vi "NGTS_DAQmx Analog Channel Scale Calibration.vi"(0 "Scale Identifier":string="Test Cal", 1 "scaled min":dbl=5.0, 2 "scaled max":dbl=1.0, 3 "scaled units":string="psi", 4 "prescaled units":string="Amps", 5 "error in":errorcluster, 6 "prescaled min":dbl=5.0, 7 "Save As Global Channel":bool, 8 "prescaled max":dbl=1.0, 9 "Author":string="Mike Ashe") -> (14 "Custom Scale Out":tag, 19 "error out":errorcluster)   [LabVIEW 2018]
doc: "Creates a new custom scale using the \"Map Ranges\" version of the \"DAQmx Create Scale (Version).vi\". It first deletes any saved scale of the same name. The Mapped Range is from Prescaled Min & Max to Scaled Min & Max. When using this method, values outside the scaled range are clipped on reads and generate an error on writes. It optionally saves the new scale to MAX.\n\nCurrently only Volts and Amps are used as Prescaled Units. \n\n2007-11 Mike Ashe\nmichael.ashe@imaginatics.net\nCell: 860-961-0876"
uses:
  <vilib>/DAQmx/create/scale.llb/DAQmx Create Scale (Linear).vi
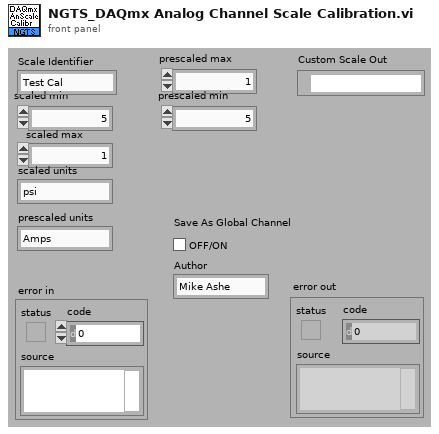
[diagram p1: front panel]
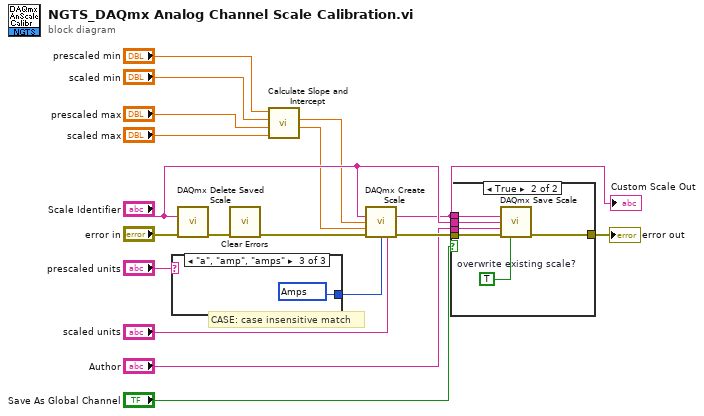
[diagram p0: block diagram]
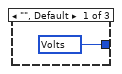
[diagram p2: hidden frame]
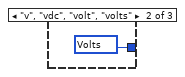
[diagram p3: hidden frame]
diagram:
  # "CASE: case insensitive match"
  n1 = case shown="\"a\", \"amp\", \"amps\"" "prescaled units" {
    tunnel: [w19 w20 w21] -> w10
    frame "", Default {
      w19 = 10348 items=["Volts"=10348, "Amps"=10342, "Deg F"=10144, "Deg C"=10143, "Deg R"=10145, "Kelvins"=10325, "Strain"=10299, "Ohms"=10384, "Hz"=10373, "Seconds"=10364, "Meters"=10219, "Inches"=10379, "Degrees"=10146, "Radians"=10273, "g"=10186, "m/s^2"=12470, "Pascals"=10081, "From TEDS"=12516] ("pre-scaled units")
    }
    frame "v", "vdc", "volt", "volts" {
      w20 = 10348 items=["Volts"=10348, "Amps"=10342, "Deg F"=10144, "Deg C"=10143, "Deg R"=10145, "Kelvins"=10325, "Strain"=10299, "Ohms"=10384, "Hz"=10373, "Seconds"=10364, "Meters"=10219, "Inches"=10379, "Degrees"=10146, "Radians"=10273, "g"=10186, "m/s^2"=12470, "Pascals"=10081, "From TEDS"=12516] ("pre-scaled units")
    }
    frame "a", "amp", "amps" {
      w21 = 10342 items=["Volts"=10348, "Amps"=10342, "Deg F"=10144, "Deg C"=10143, "Deg R"=10145, "Kelvins"=10325, "Strain"=10299, "Ohms"=10384, "Hz"=10373, "Seconds"=10364, "Meters"=10219, "Inches"=10379, "Degrees"=10146, "Radians"=10273, "g"=10186, "m/s^2"=12470, "Pascals"=10081, "From TEDS"=12516] ("pre-scaled units")
    }
  }
  n2 = call <vilib>:"DAQmx Delete Saved Scale.vi"("scale name"="Scale Identifier", "error in"="error in") -> ("error out"=w9:errorcluster)  [unwired: 13 in]
  n3 = call <vilib>:"Clear Errors.vi"("error in (no error)"=w9) -> ("error out"=w7:errorcluster)  [unwired: 5 in, 1 out]
  n4 = call "Calculate Slope and Intercept.vi"("y2"="scaled max", "x2"="prescaled max", "y1"="scaled min", "x1"="prescaled min") -> ("y-intercept"=w1:dbl, "slope"=w2:dbl)  [unwired: 6 in]
  n5 = call-poly <vilib>:"DAQmx Create Scale.vi"("name"="Scale Identifier", "slope"=w2, "y-intercept"=w1, "error in"=w7, "pre-scaled units"=w10, "scaled units"="scaled units") -> ("scale out"=w13:tag, "error out"=w18:errorcluster)  [unwired: 8 in]
  "Custom Scale Out" <- w13
  n6 = case shown="True" "Save As Global Channel" {
    tunnel: w13 -> [_ w28]
    tunnel: w18 -> [w22 w27]
    tunnel: "Author" -> [_ w26]
    tunnel: "Scale Identifier" -> [_ w25]
    tunnel: [w22 w24] -> w14
    frame False {
    }
    frame True {
      w23 = TRUE  # overwrite existing scale?
      n7 = call <vilib>:"DAQmx Save Scale.vi"("scale name"=w28, "save as"=w25, "author"=w26, "error in"=w27, "overwrite existing scale?"=w23) -> ("error out"=w24:errorcluster)  [unwired: 10 in]
    }
  }
  "error out" <- w14
